vi "Auton-MoveDistance.vi"(10 "Distance":dbl) -> (2 "Done?":bool)   [LabVIEW 2014]
uses:
  Robot Global Data.vi
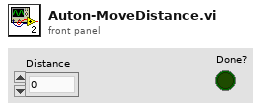
[diagram p1: front panel]
types:
  T1 = typedef "WPI_EncoderDevRef.ctl" = cluster{"DevStatus":errorcluster, "EncoderIndex":T2, "CounterIndex":T3, "DistancePerCount":dbl, "Decoding Type":T4}
  T2 = typedef "FPGA_EncoderIdx.ctl" = enum8{"Enc 0", "Enc 1", "Enc 2", "Enc 3", "Enc 4", "Enc 5", "Enc 6", "Enc 7", "Invalid"}
  T3 = typedef "FPGA_CounterCtrSystemIndex.ctl" = enum8{"Ctr 0", "Ctr 1", "Ctr 2", "Ctr 3", "Ctr 4", "Ctr 5", "Ctr 6", "Ctr 7", "Invalid"}
  T4 = typedef "WPI_EncoderType.ctl" = enum16{"1x", "2x", "4x"}
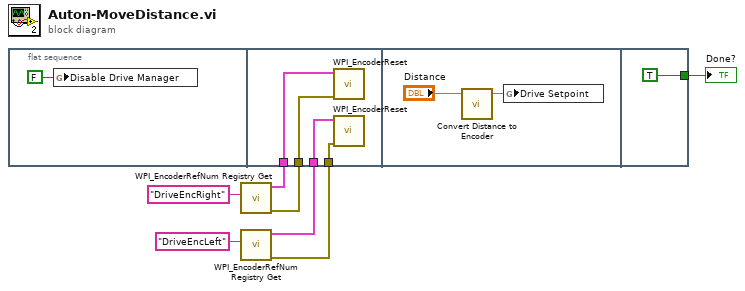
[diagram p0: block diagram]
diagram:
  n1 = flat-sequence {
    tunnel: w4 -> [w11]
    tunnel: w3 -> [w12]
    tunnel: w2 -> [w10]
    tunnel: w1 -> [w9]
    tunnel: [TRUE] -> w7
    frame #0 {
      n2 = global write "Robot Global Data.vi" "Disable Drive Manager"(FALSE) -> ()
    }
    frame #1 {
      n3 = call <vilib>:"WPI_EncoderReset.vi"("error in (no error)"=w10, "EncoderDevRef"=w9) -> ()  [unwired: 8 in, 2 out]
      n4 = call <vilib>:"WPI_EncoderReset.vi"("error in (no error)"=w12, "EncoderDevRef"=w11) -> ()  [unwired: 8 in, 2 out]
    }
    frame #2 {
      n5 = call "Convert Distance to Encoder.vi"("Dist (ft)"="Distance") -> ("Encoder"=w14:dbl)  [unwired: 4 in]
      n6 = global write "Robot Global Data.vi" "Drive Setpoint"(w14) -> ()
    }
    frame #3 {
    }
  }
  n7 = call <vilib>:"WPI_EncoderRefNum Registry Get.vi"("refnum name"="DriveEncRight") -> ("error out"=w2:errorcluster, "EncoderDevRef"=w1:T1)  [unwired: 9 in]
  n8 = call <vilib>:"WPI_EncoderRefNum Registry Get.vi"("refnum name"="DriveEncLeft") -> ("error out"=w3:errorcluster, "EncoderDevRef"=w4:T1)  [unwired: 9 in]
  "Done?" <- w7
